vi "SRsesnsitivityConversion5210.vi"(9 "Sen":dbl format="%#_13g", 11 "Input":dbl=0.00012) -> (3 "Output":dbl=0.00012)   [LabVIEW 2013]
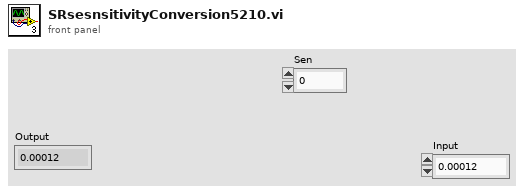
[diagram p1: front panel]
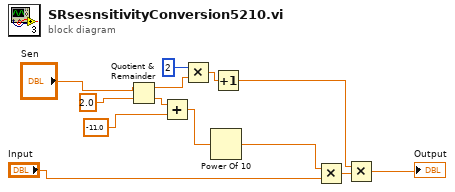
[diagram p0: block diagram]
diagram:
  n1 = Quotient & Remainder(x="Sen", y=2.0) -> (x-y*floor(x/y)=w3:dbl, floor(x/y)=w11:dbl)
  n2 = Add(x=w11, y=-11.0) -> (x+y=w9:dbl)
  n3 = Multiply(x=2, y=w3) -> (x*y=w2:dbl)
  n4 = Power Of 10(x=w9) -> (10^x=w8:dbl)
  n5 = Increment(x=w2) -> (x+1=w5:dbl)
  n6 = Multiply(x=w8, y="Input") -> (x*y=w6:dbl)
  n7 = Multiply(x=w5, y=w6) -> (x*y=→"Output":dbl)
